vi "carica dati prove.vi"(4 "Riga selezionata":i32, 6 "TIPO COLLEGAMENTO":u16, 7 "Carica tabelle?":bool, 8 "Dati in":string[][](array[string]), 9 "Tabella":i32, 10 "prova":string, 11 "Dati prove in":T1) -> (0 "Per tabella":string[][](array[string]), 1 "Riga selezionata":string[](array[string]), 3 "Dati prove out":T1)   [LabVIEW 2019]
uses:
  TypeDef/Dati collaudo.ctl
panel:
  out "x-y":u32
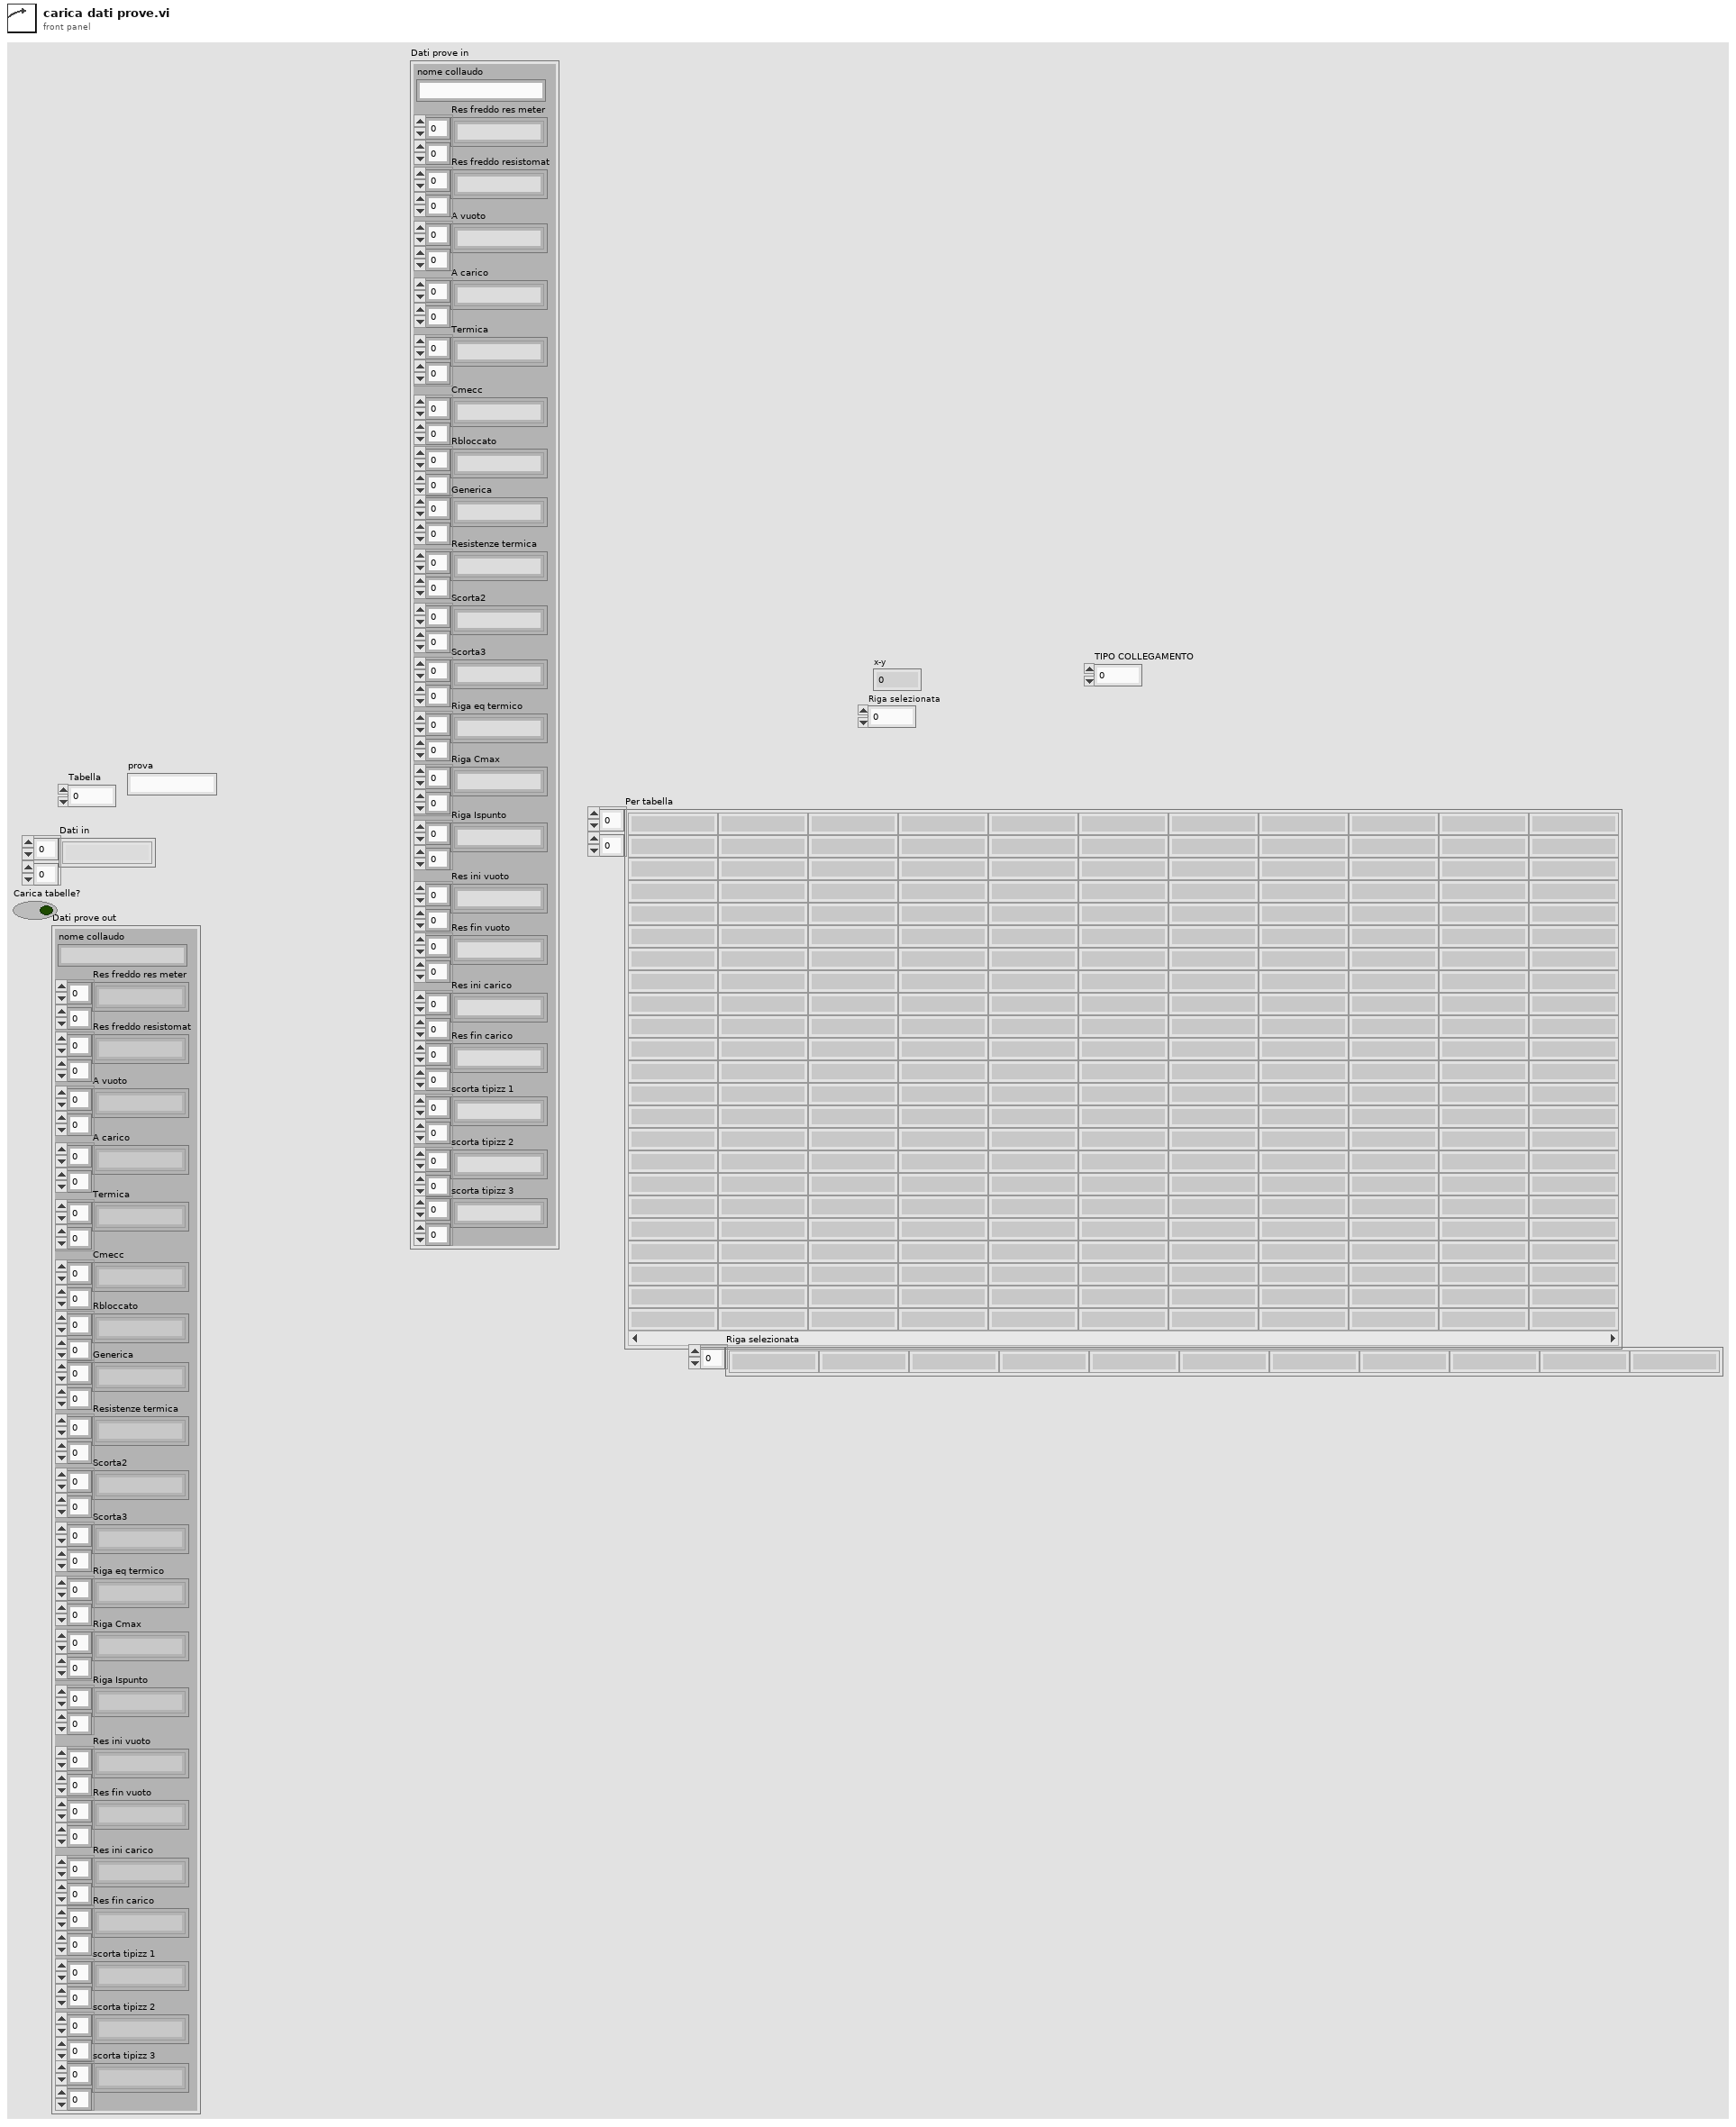
[diagram p1: front panel]
types:
  T1 = typedef "Dati collaudo.ctl" = cluster{"nome collaudo":string, "Res freddo res meter":string[][], "Res freddo resistomat":string[][], "A vuoto":string[][], "A carico":string[][], "Termica":string[][], "Cmecc":string[][], "Rbloccato":string[][], "Generica":string[][], "Resistenze termica":string[][], "Scorta2":string[][], "Scorta3":string[][], "Riga eq termico":string[][], "Riga Cmax":string[][], "Riga Ispunto":string[][], "Res ini vuoto":string[][], "Res fin vuoto":string[][], "Res ini carico":string[][], "Res fin carico":string[][], "scorta tipizz 1":string[][], "scorta tipizz 2":string[][], "scorta tipizz 3":string[][]}
  T2 = cluster{"Nome":string, "TAB":cluster{"Visibile ?":bool, "Salva?":bool}, "decimali":i8, "Medie RT":i8}[]
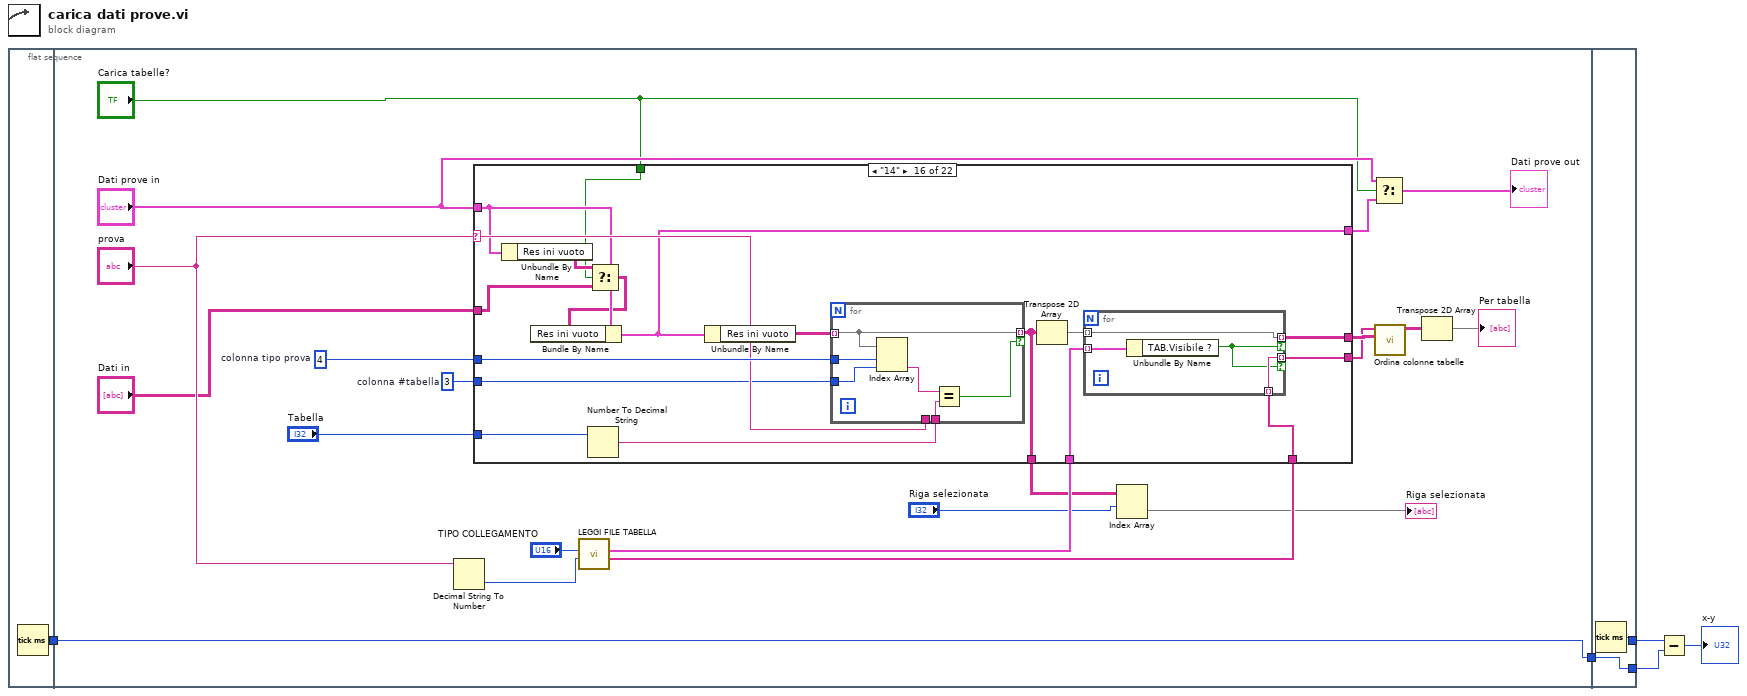
[diagram p0: block diagram]
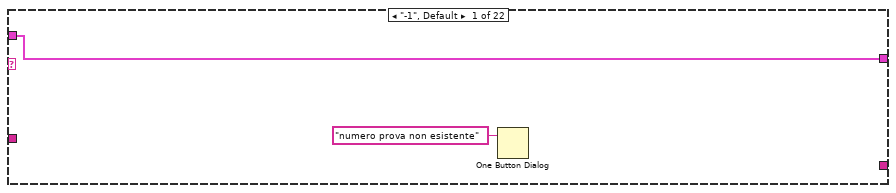
[diagram p2: hidden frame]
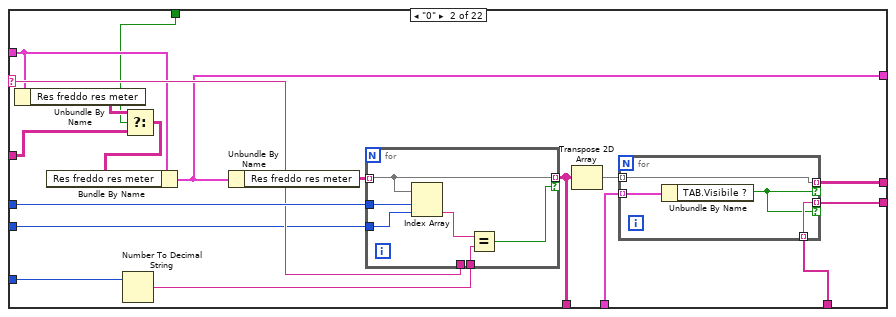
[diagram p3: hidden frame]
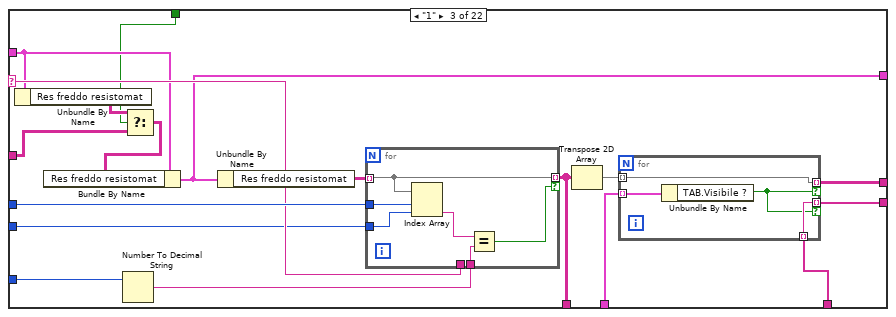
[diagram p4: hidden frame]
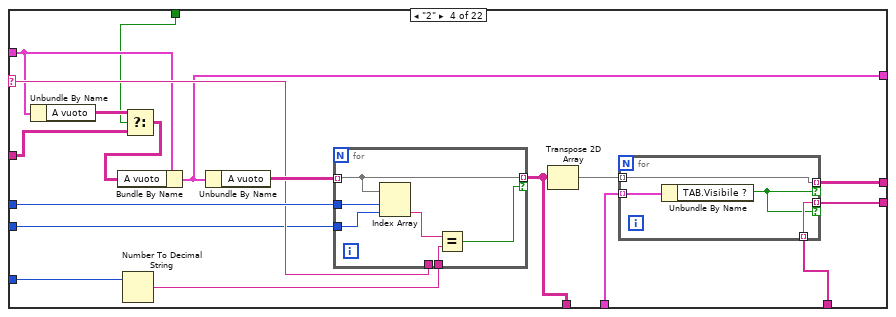
[diagram p5: hidden frame]
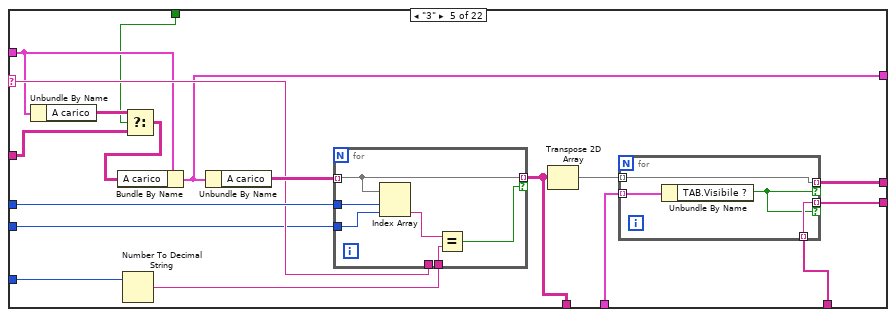
[diagram p6: hidden frame]
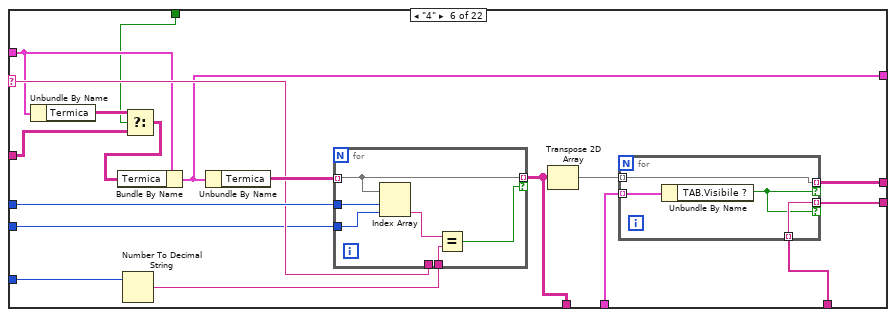
[diagram p7: hidden frame]
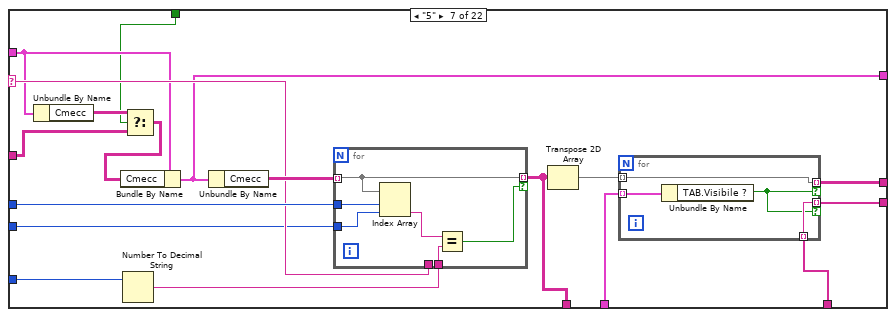
[diagram p8: hidden frame]
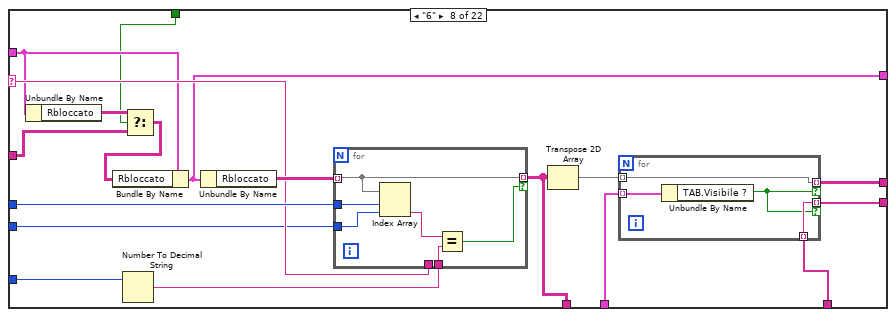
[diagram p9: hidden frame]
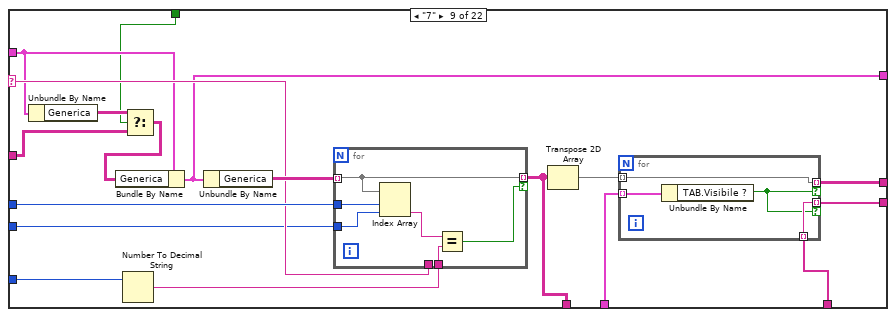
[diagram p10: hidden frame]
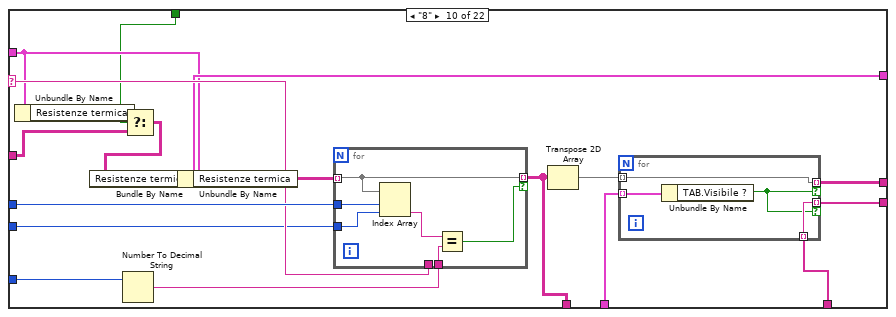
[diagram p11: hidden frame]
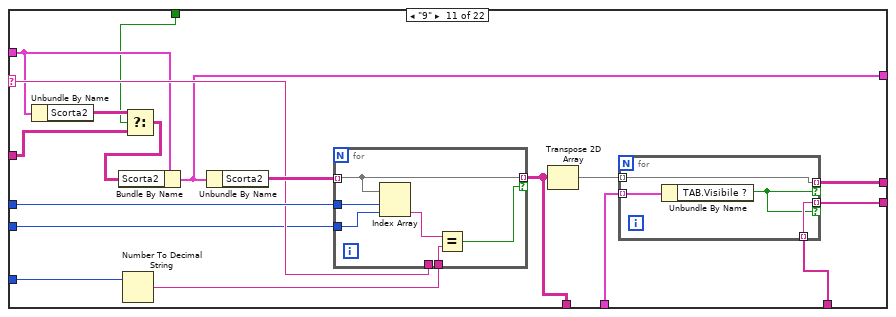
[diagram p12: hidden frame]
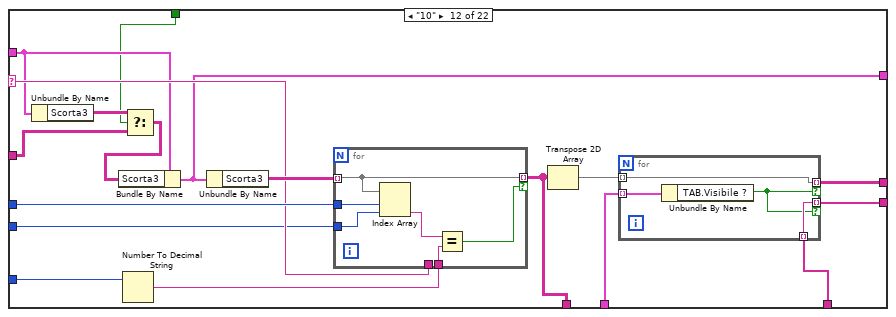
[diagram p13: hidden frame]
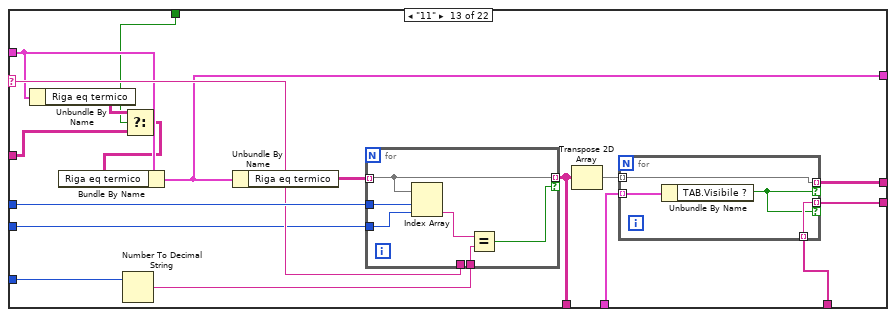
[diagram p14: hidden frame]
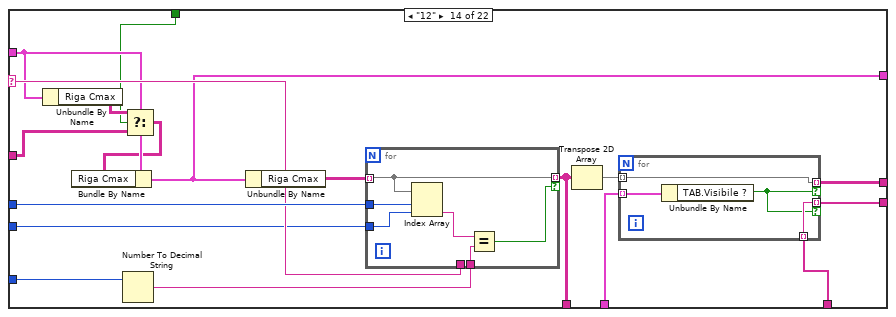
[diagram p15: hidden frame]
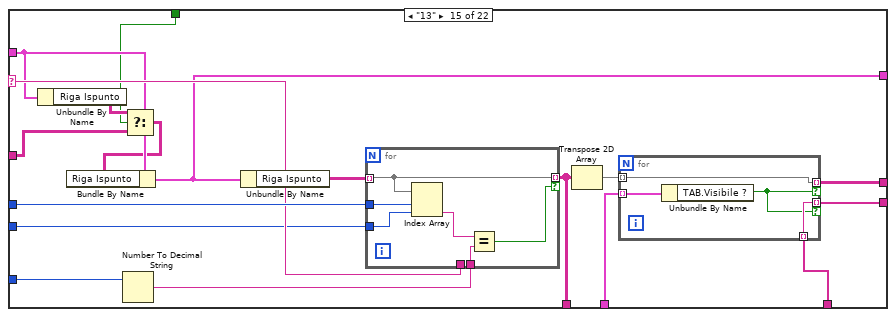
[diagram p16: hidden frame]
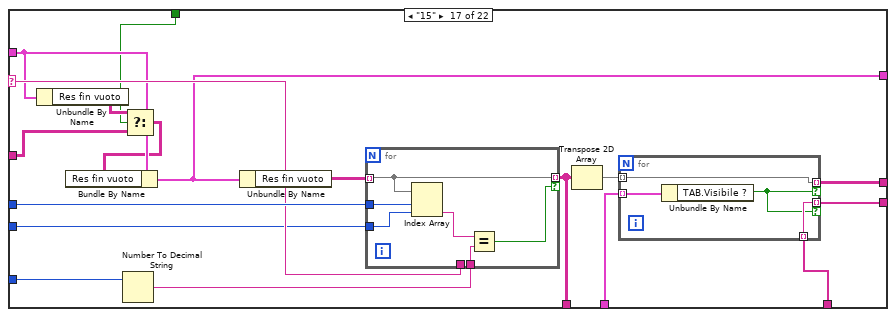
[diagram p17: hidden frame]
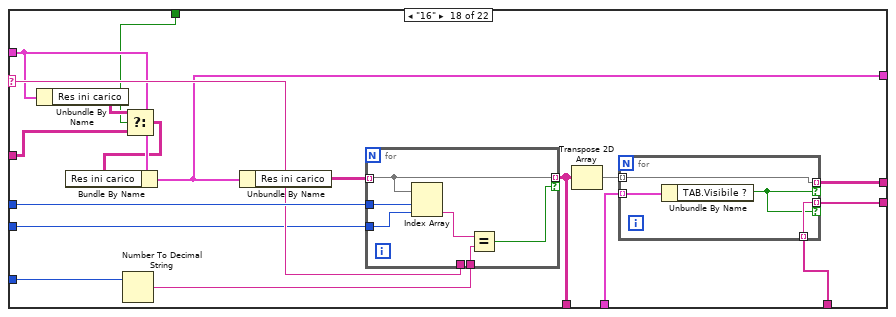
[diagram p18: hidden frame]
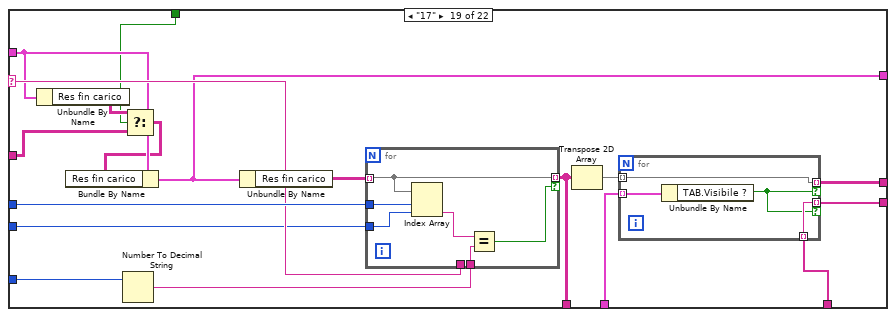
[diagram p19: hidden frame]
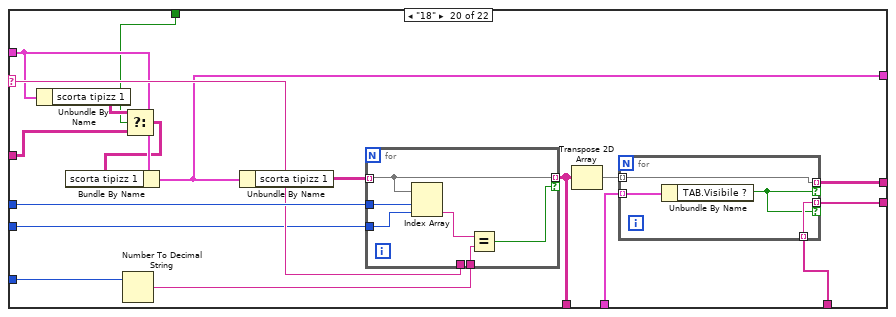
[diagram p20: hidden frame]
diagram:
  n1 = flat-sequence {
    tunnel: [w6] -> w2
    tunnel: [w13] -> w3
    tunnel: w2 -> [w13]
    tunnel: [w619] -> w5
    tunnel: [w618] -> w4
    tunnel: w3 -> [w618]
    frame #0 {
      n2 = Tick Count (ms)() -> (millisecond timer value=w6:u32)
    }
    frame #1 {
      w19 = 3  # colonna #tabella
      w20 = 4  # colonna tipo prova
      n3 = Decimal String To Number(string="prova") -> (number=w14:i32)  [unwired: 2 in, 1 out]
      n4 = call "LEGGI FILE TABELLA.vi"("INDICE TABELLA"=w14, "TIPO COLLEGAMENTO"="TIPO COLLEGAMENTO") -> ("Array INDICI"=w16:string[], "Array"=w17:T2)  [unwired: 7 in, 1 out]
      n5 = case shown="\"14\"" "prova" {
        selector: "prova" -> [_ w41 w69 w97 w125 w153 w181 w209 w237 w265 w293 w321 w349 w377 w405 w433 w461 w489 w517 w545 w573 w601]
        tunnel: "Dati prove in" -> [w29 w34 w62 w90 w118 w146 w174 w202 w230 w258 w286 w314 w342 w370 w398 w426 w454 w482 w510 w538 w566 w594]
        tunnel: [w29 w40 w68 w96 w124 w152 w180 w208 w236 w264 w292 w320 w348 w376 w404 w432 w460 w488 w516 w544 w572 w600] -> w26
        tunnel: "Tabella" -> [_ w39 w67 w95 w123 w151 w179 w207 w235 w263 w291 w319 w347 w375 w403 w431 w459 w487 w515 w543 w571 w599]
        tunnel: [_ w47 w75 w103 w131 w159 w187 w215 w243 w271 w299 w327 w355 w383 w411 w439 w467 w495 w523 w551 w579 w607] -> w23
        tunnel: w16 -> [_ w45 w73 w101 w129 w157 w185 w213 w241 w269 w297 w325 w353 w381 w409 w437 w465 w493 w521 w549 w577 w605]
        tunnel: [_ w44 w72 w100 w128 w156 w184 w212 w240 w268 w296 w324 w352 w380 w408 w436 w464 w492 w520 w548 w576 w604] -> w21
        tunnel: w20 -> [_ w42 w70 w98 w126 w154 w182 w210 w238 w266 w294 w322 w350 w378 w406 w434 w462 w490 w518 w546 w574 w602]
        tunnel: w19 -> [_ w38 w66 w94 w122 w150 w178 w206 w234 w262 w290 w318 w346 w374 w402 w430 w458 w486 w514 w542 w570 w598]
        tunnel: w17 -> [_ w36 w64 w92 w120 w148 w176 w204 w232 w260 w288 w316 w344 w372 w400 w428 w456 w484 w512 w540 w568 w596]
        tunnel: "Carica tabelle?" -> [_ w32 w60 w88 w116 w144 w172 w200 w228 w256 w284 w312 w340 w368 w396 w424 w452 w480 w508 w536 w564 w592]
        tunnel: "Dati in" -> [_ w33 w61 w89 w117 w145 w173 w201 w229 w257 w285 w313 w341 w369 w397 w425 w453 w481 w509 w537 w565 w593]
        tunnel: [_ w30 w58 w86 w114 w142 w170 w198 w226 w254 w282 w310 w338 w366 w394 w422 w450 w478 w506 w534 w562 w590] -> w9
        frame "-1", Default {
          n6 = One Button Dialog(message="numero prova non esistente") -> ()  [unwired: 1 in, 1 out]
        }
        frame "0" {
          n7 = Unbundle By Name(w34) -> ("Res freddo res meter"=w35:string[][])
          n8 = Number To Decimal String(number=w39) -> (decimal integer string=w37:string)  [unwired: 1 in]
          n9 = Select(t=w35, s=w32, f=w33) -> (s? t:f=w31:string[][])
          n10 = Bundle By Name(cluster=w34, "Res freddo res meter"=w31) -> (w40:T1)
          n11 = Unbundle By Name(w40) -> ("Res freddo res meter"=w43:string[][])
          n12 = for {
            tunnel: w43 -> [w52] mode=indexing
            tunnel: [w52] -> w30 mode=indexing if=w48
            tunnel: w42 -> [w53]
            tunnel: w41 -> [_]
            tunnel: w38 -> [w51]
            tunnel: w37 -> [w49]
            n13 = Index Array(array=w52, index #1=w53, index #2=w51) -> (element #2=w50:string)  [unwired: 1 out]
            n14 = Equal?(x=w50, y=w49) -> (x = y?=w48:bool)
          }
          n15 = Transpose 2D Array(2D array=w30) -> (transposed array=w46:string[][])
          n16 = for {
            tunnel: w46 -> [w57] mode=indexing
            tunnel: [w57] -> w47 mode=indexing if=w54
            tunnel: w36 -> [w56] mode=indexing
            tunnel: [w55] -> w44 mode=indexing if=w54
            tunnel: w45 -> [w55] mode=indexing
            n17 = Unbundle By Name(w56) -> ("TAB.Visibile ?"=w54:bool)
          }
        }
        frame "1" {
          n18 = Unbundle By Name(w62) -> ("Res freddo resistomat"=w63:string[][])
          n19 = Number To Decimal String(number=w67) -> (decimal integer string=w65:string)  [unwired: 1 in]
          n20 = Select(t=w63, s=w60, f=w61) -> (s? t:f=w59:string[][])
          n21 = Bundle By Name(cluster=w62, "Res freddo resistomat"=w59) -> (w68:T1)
          n22 = Unbundle By Name(w68) -> ("Res freddo resistomat"=w71:string[][])
          n23 = for {
            tunnel: w71 -> [w80] mode=indexing
            tunnel: [w80] -> w58 mode=indexing if=w76
            tunnel: w70 -> [w81]
            tunnel: w69 -> [_]
            tunnel: w66 -> [w79]
            tunnel: w65 -> [w77]
            n24 = Index Array(array=w80, index #1=w81, index #2=w79) -> (element #2=w78:string)  [unwired: 1 out]
            n25 = Equal?(x=w78, y=w77) -> (x = y?=w76:bool)
          }
          n26 = Transpose 2D Array(2D array=w58) -> (transposed array=w74:string[][])
          n27 = for {
            tunnel: w74 -> [w85] mode=indexing
            tunnel: [w85] -> w75 mode=indexing if=w82
            tunnel: w64 -> [w84] mode=indexing
            tunnel: [w83] -> w72 mode=indexing if=w82
            tunnel: w73 -> [w83] mode=indexing
            n28 = Unbundle By Name(w84) -> ("TAB.Visibile ?"=w82:bool)
          }
        }
        frame "2" {
          n29 = Unbundle By Name(w90) -> ("A vuoto"=w91:string[][])
          n30 = Number To Decimal String(number=w95) -> (decimal integer string=w93:string)  [unwired: 1 in]
          n31 = Select(t=w91, s=w88, f=w89) -> (s? t:f=w87:string[][])
          n32 = Bundle By Name(cluster=w90, "A vuoto"=w87) -> (w96:T1)
          n33 = Unbundle By Name(w96) -> ("A vuoto"=w99:string[][])
          n34 = for {
            tunnel: w99 -> [w108] mode=indexing
            tunnel: [w108] -> w86 mode=indexing if=w104
            tunnel: w98 -> [w109]
            tunnel: w97 -> [_]
            tunnel: w94 -> [w107]
            tunnel: w93 -> [w105]
            n35 = Index Array(array=w108, index #1=w109, index #2=w107) -> (element #2=w106:string)  [unwired: 1 out]
            n36 = Equal?(x=w106, y=w105) -> (x = y?=w104:bool)
          }
          n37 = Transpose 2D Array(2D array=w86) -> (transposed array=w102:string[][])
          n38 = for {
            tunnel: w102 -> [w113] mode=indexing
            tunnel: [w113] -> w103 mode=indexing if=w110
            tunnel: w92 -> [w112] mode=indexing
            tunnel: [w111] -> w100 mode=indexing if=w110
            tunnel: w101 -> [w111] mode=indexing
            n39 = Unbundle By Name(w112) -> ("TAB.Visibile ?"=w110:bool)
          }
        }
        frame "3" {
          n40 = Unbundle By Name(w118) -> ("A carico"=w119:string[][])
          n41 = Number To Decimal String(number=w123) -> (decimal integer string=w121:string)  [unwired: 1 in]
          n42 = Select(t=w119, s=w116, f=w117) -> (s? t:f=w115:string[][])
          n43 = Bundle By Name(cluster=w118, "A carico"=w115) -> (w124:T1)
          n44 = Unbundle By Name(w124) -> ("A carico"=w127:string[][])
          n45 = for {
            tunnel: w127 -> [w136] mode=indexing
            tunnel: [w136] -> w114 mode=indexing if=w132
            tunnel: w126 -> [w137]
            tunnel: w125 -> [_]
            tunnel: w122 -> [w135]
            tunnel: w121 -> [w133]
            n46 = Index Array(array=w136, index #1=w137, index #2=w135) -> (element #2=w134:string)  [unwired: 1 out]
            n47 = Equal?(x=w134, y=w133) -> (x = y?=w132:bool)
          }
          n48 = Transpose 2D Array(2D array=w114) -> (transposed array=w130:string[][])
          n49 = for {
            tunnel: w130 -> [w141] mode=indexing
            tunnel: [w141] -> w131 mode=indexing if=w138
            tunnel: w120 -> [w140] mode=indexing
            tunnel: [w139] -> w128 mode=indexing if=w138
            tunnel: w129 -> [w139] mode=indexing
            n50 = Unbundle By Name(w140) -> ("TAB.Visibile ?"=w138:bool)
          }
        }
        frame "4" {
          n51 = Unbundle By Name(w146) -> ("Termica"=w147:string[][])
          n52 = Number To Decimal String(number=w151) -> (decimal integer string=w149:string)  [unwired: 1 in]
          n53 = Select(t=w147, s=w144, f=w145) -> (s? t:f=w143:string[][])
          n54 = Bundle By Name(cluster=w146, "Termica"=w143) -> (w152:T1)
          n55 = Unbundle By Name(w152) -> ("Termica"=w155:string[][])
          n56 = for {
            tunnel: w155 -> [w164] mode=indexing
            tunnel: [w164] -> w142 mode=indexing if=w160
            tunnel: w154 -> [w165]
            tunnel: w153 -> [_]
            tunnel: w150 -> [w163]
            tunnel: w149 -> [w161]
            n57 = Index Array(array=w164, index #1=w165, index #2=w163) -> (element #2=w162:string)  [unwired: 1 out]
            n58 = Equal?(x=w162, y=w161) -> (x = y?=w160:bool)
          }
          n59 = Transpose 2D Array(2D array=w142) -> (transposed array=w158:string[][])
          n60 = for {
            tunnel: w158 -> [w169] mode=indexing
            tunnel: [w169] -> w159 mode=indexing if=w166
            tunnel: w148 -> [w168] mode=indexing
            tunnel: [w167] -> w156 mode=indexing if=w166
            tunnel: w157 -> [w167] mode=indexing
            n61 = Unbundle By Name(w168) -> ("TAB.Visibile ?"=w166:bool)
          }
        }
        frame "5" {
          n62 = Unbundle By Name(w174) -> ("Cmecc"=w175:string[][])
          n63 = Number To Decimal String(number=w179) -> (decimal integer string=w177:string)  [unwired: 1 in]
          n64 = Select(t=w175, s=w172, f=w173) -> (s? t:f=w171:string[][])
          n65 = Bundle By Name(cluster=w174, "Cmecc"=w171) -> (w180:T1)
          n66 = Unbundle By Name(w180) -> ("Cmecc"=w183:string[][])
          n67 = for {
            tunnel: w183 -> [w192] mode=indexing
            tunnel: [w192] -> w170 mode=indexing if=w188
            tunnel: w182 -> [w193]
            tunnel: w181 -> [_]
            tunnel: w178 -> [w191]
            tunnel: w177 -> [w189]
            n68 = Index Array(array=w192, index #1=w193, index #2=w191) -> (element #2=w190:string)  [unwired: 1 out]
            n69 = Equal?(x=w190, y=w189) -> (x = y?=w188:bool)
          }
          n70 = Transpose 2D Array(2D array=w170) -> (transposed array=w186:string[][])
          n71 = for {
            tunnel: w186 -> [w197] mode=indexing
            tunnel: [w197] -> w187 mode=indexing if=w194
            tunnel: w176 -> [w196] mode=indexing
            tunnel: [w195] -> w184 mode=indexing if=w194
            tunnel: w185 -> [w195] mode=indexing
            n72 = Unbundle By Name(w196) -> ("TAB.Visibile ?"=w194:bool)
          }
        }
        frame "6" {
          n73 = Unbundle By Name(w202) -> ("Rbloccato"=w203:string[][])
          n74 = Number To Decimal String(number=w207) -> (decimal integer string=w205:string)  [unwired: 1 in]
          n75 = Select(t=w203, s=w200, f=w201) -> (s? t:f=w199:string[][])
          n76 = Bundle By Name(cluster=w202, "Rbloccato"=w199) -> (w208:T1)
          n77 = Unbundle By Name(w208) -> ("Rbloccato"=w211:string[][])
          n78 = for {
            tunnel: w211 -> [w220] mode=indexing
            tunnel: [w220] -> w198 mode=indexing if=w216
            tunnel: w210 -> [w221]
            tunnel: w209 -> [_]
            tunnel: w206 -> [w219]
            tunnel: w205 -> [w217]
            n79 = Index Array(array=w220, index #1=w221, index #2=w219) -> (element #2=w218:string)  [unwired: 1 out]
            n80 = Equal?(x=w218, y=w217) -> (x = y?=w216:bool)
          }
          n81 = Transpose 2D Array(2D array=w198) -> (transposed array=w214:string[][])
          n82 = for {
            tunnel: w214 -> [w225] mode=indexing
            tunnel: [w225] -> w215 mode=indexing if=w222
            tunnel: w204 -> [w224] mode=indexing
            tunnel: [w223] -> w212 mode=indexing if=w222
            tunnel: w213 -> [w223] mode=indexing
            n83 = Unbundle By Name(w224) -> ("TAB.Visibile ?"=w222:bool)
          }
        }
        frame "7" {
          n84 = Unbundle By Name(w230) -> ("Generica"=w231:string[][])
          n85 = Number To Decimal String(number=w235) -> (decimal integer string=w233:string)  [unwired: 1 in]
          n86 = Select(t=w231, s=w228, f=w229) -> (s? t:f=w227:string[][])
          n87 = Bundle By Name(cluster=w230, "Generica"=w227) -> (w236:T1)
          n88 = Unbundle By Name(w236) -> ("Generica"=w239:string[][])
          n89 = for {
            tunnel: w239 -> [w248] mode=indexing
            tunnel: [w248] -> w226 mode=indexing if=w244
            tunnel: w238 -> [w249]
            tunnel: w237 -> [_]
            tunnel: w234 -> [w247]
            tunnel: w233 -> [w245]
            n90 = Index Array(array=w248, index #1=w249, index #2=w247) -> (element #2=w246:string)  [unwired: 1 out]
            n91 = Equal?(x=w246, y=w245) -> (x = y?=w244:bool)
          }
          n92 = Transpose 2D Array(2D array=w226) -> (transposed array=w242:string[][])
          n93 = for {
            tunnel: w242 -> [w253] mode=indexing
            tunnel: [w253] -> w243 mode=indexing if=w250
            tunnel: w232 -> [w252] mode=indexing
            tunnel: [w251] -> w240 mode=indexing if=w250
            tunnel: w241 -> [w251] mode=indexing
            n94 = Unbundle By Name(w252) -> ("TAB.Visibile ?"=w250:bool)
          }
        }
        frame "8" {
          n95 = Unbundle By Name(w258) -> ("Resistenze termica"=w259:string[][])
          n96 = Number To Decimal String(number=w263) -> (decimal integer string=w261:string)  [unwired: 1 in]
          n97 = Select(t=w259, s=w256, f=w257) -> (s? t:f=w255:string[][])
          n98 = Bundle By Name(cluster=w258, "Resistenze termica"=w255) -> (w264:T1)
          n99 = Unbundle By Name(w264) -> ("Resistenze termica"=w267:string[][])
          n100 = for {
            tunnel: w267 -> [w276] mode=indexing
            tunnel: [w276] -> w254 mode=indexing if=w272
            tunnel: w266 -> [w277]
            tunnel: w265 -> [_]
            tunnel: w262 -> [w275]
            tunnel: w261 -> [w273]
            n101 = Index Array(array=w276, index #1=w277, index #2=w275) -> (element #2=w274:string)  [unwired: 1 out]
            n102 = Equal?(x=w274, y=w273) -> (x = y?=w272:bool)
          }
          n103 = Transpose 2D Array(2D array=w254) -> (transposed array=w270:string[][])
          n104 = for {
            tunnel: w270 -> [w281] mode=indexing
            tunnel: [w281] -> w271 mode=indexing if=w278
            tunnel: w260 -> [w280] mode=indexing
            tunnel: [w279] -> w268 mode=indexing if=w278
            tunnel: w269 -> [w279] mode=indexing
            n105 = Unbundle By Name(w280) -> ("TAB.Visibile ?"=w278:bool)
          }
        }
        frame "9" {
          n106 = Unbundle By Name(w286) -> ("Scorta2"=w287:string[][])
          n107 = Number To Decimal String(number=w291) -> (decimal integer string=w289:string)  [unwired: 1 in]
          n108 = Select(t=w287, s=w284, f=w285) -> (s? t:f=w283:string[][])
          n109 = Bundle By Name(cluster=w286, "Scorta2"=w283) -> (w292:T1)
          n110 = Unbundle By Name(w292) -> ("Scorta2"=w295:string[][])
          n111 = for {
            tunnel: w295 -> [w304] mode=indexing
            tunnel: [w304] -> w282 mode=indexing if=w300
            tunnel: w294 -> [w305]
            tunnel: w293 -> [_]
            tunnel: w290 -> [w303]
            tunnel: w289 -> [w301]
            n112 = Index Array(array=w304, index #1=w305, index #2=w303) -> (element #2=w302:string)  [unwired: 1 out]
            n113 = Equal?(x=w302, y=w301) -> (x = y?=w300:bool)
          }
          n114 = Transpose 2D Array(2D array=w282) -> (transposed array=w298:string[][])
          n115 = for {
            tunnel: w298 -> [w309] mode=indexing
            tunnel: [w309] -> w299 mode=indexing if=w306
            tunnel: w288 -> [w308] mode=indexing
            tunnel: [w307] -> w296 mode=indexing if=w306
            tunnel: w297 -> [w307] mode=indexing
            n116 = Unbundle By Name(w308) -> ("TAB.Visibile ?"=w306:bool)
          }
        }
        frame "10" {
          n117 = Unbundle By Name(w314) -> ("Scorta3"=w315:string[][])
          n118 = Number To Decimal String(number=w319) -> (decimal integer string=w317:string)  [unwired: 1 in]
          n119 = Select(t=w315, s=w312, f=w313) -> (s? t:f=w311:string[][])
          n120 = Bundle By Name(cluster=w314, "Scorta3"=w311) -> (w320:T1)
          n121 = Unbundle By Name(w320) -> ("Scorta3"=w323:string[][])
          n122 = for {
            tunnel: w323 -> [w332] mode=indexing
            tunnel: [w332] -> w310 mode=indexing if=w328
            tunnel: w322 -> [w333]
            tunnel: w321 -> [_]
            tunnel: w318 -> [w331]
            tunnel: w317 -> [w329]
            n123 = Index Array(array=w332, index #1=w333, index #2=w331) -> (element #2=w330:string)  [unwired: 1 out]
            n124 = Equal?(x=w330, y=w329) -> (x = y?=w328:bool)
          }
          n125 = Transpose 2D Array(2D array=w310) -> (transposed array=w326:string[][])
          n126 = for {
            tunnel: w326 -> [w337] mode=indexing
            tunnel: [w337] -> w327 mode=indexing if=w334
            tunnel: w316 -> [w336] mode=indexing
            tunnel: [w335] -> w324 mode=indexing if=w334
            tunnel: w325 -> [w335] mode=indexing
            n127 = Unbundle By Name(w336) -> ("TAB.Visibile ?"=w334:bool)
          }
        }
        frame "11" {
          n128 = Unbundle By Name(w342) -> ("Riga eq termico"=w343:string[][])
          n129 = Number To Decimal String(number=w347) -> (decimal integer string=w345:string)  [unwired: 1 in]
          n130 = Select(t=w343, s=w340, f=w341) -> (s? t:f=w339:string[][])
          n131 = Bundle By Name(cluster=w342, "Riga eq termico"=w339) -> (w348:T1)
          n132 = Unbundle By Name(w348) -> ("Riga eq termico"=w351:string[][])
          n133 = for {
            tunnel: w351 -> [w360] mode=indexing
            tunnel: [w360] -> w338 mode=indexing if=w356
            tunnel: w350 -> [w361]
            tunnel: w349 -> [_]
            tunnel: w346 -> [w359]
            tunnel: w345 -> [w357]
            n134 = Index Array(array=w360, index #1=w361, index #2=w359) -> (element #2=w358:string)  [unwired: 1 out]
            n135 = Equal?(x=w358, y=w357) -> (x = y?=w356:bool)
          }
          n136 = Transpose 2D Array(2D array=w338) -> (transposed array=w354:string[][])
          n137 = for {
            tunnel: w354 -> [w365] mode=indexing
            tunnel: [w365] -> w355 mode=indexing if=w362
            tunnel: w344 -> [w364] mode=indexing
            tunnel: [w363] -> w352 mode=indexing if=w362
            tunnel: w353 -> [w363] mode=indexing
            n138 = Unbundle By Name(w364) -> ("TAB.Visibile ?"=w362:bool)
          }
        }
        frame "12" {
          n139 = Unbundle By Name(w370) -> ("Riga Cmax"=w371:string[][])
          n140 = Number To Decimal String(number=w375) -> (decimal integer string=w373:string)  [unwired: 1 in]
          n141 = Select(t=w371, s=w368, f=w369) -> (s? t:f=w367:string[][])
          n142 = Bundle By Name(cluster=w370, "Riga Cmax"=w367) -> (w376:T1)
          n143 = Unbundle By Name(w376) -> ("Riga Cmax"=w379:string[][])
          n144 = for {
            tunnel: w379 -> [w388] mode=indexing
            tunnel: [w388] -> w366 mode=indexing if=w384
            tunnel: w378 -> [w389]
            tunnel: w377 -> [_]
            tunnel: w374 -> [w387]
            tunnel: w373 -> [w385]
            n145 = Index Array(array=w388, index #1=w389, index #2=w387) -> (element #2=w386:string)  [unwired: 1 out]
            n146 = Equal?(x=w386, y=w385) -> (x = y?=w384:bool)
          }
          n147 = Transpose 2D Array(2D array=w366) -> (transposed array=w382:string[][])
          n148 = for {
            tunnel: w382 -> [w393] mode=indexing
            tunnel: [w393] -> w383 mode=indexing if=w390
            tunnel: w372 -> [w392] mode=indexing
            tunnel: [w391] -> w380 mode=indexing if=w390
            tunnel: w381 -> [w391] mode=indexing
            n149 = Unbundle By Name(w392) -> ("TAB.Visibile ?"=w390:bool)
          }
        }
        frame "13" {
          n150 = Unbundle By Name(w398) -> ("Riga Ispunto"=w399:string[][])
          n151 = Number To Decimal String(number=w403) -> (decimal integer string=w401:string)  [unwired: 1 in]
          n152 = Select(t=w399, s=w396, f=w397) -> (s? t:f=w395:string[][])
          n153 = Bundle By Name(cluster=w398, "Riga Ispunto"=w395) -> (w404:T1)
          n154 = Unbundle By Name(w404) -> ("Riga Ispunto"=w407:string[][])
          n155 = for {
            tunnel: w407 -> [w416] mode=indexing
            tunnel: [w416] -> w394 mode=indexing if=w412
            tunnel: w406 -> [w417]
            tunnel: w405 -> [_]
            tunnel: w402 -> [w415]
            tunnel: w401 -> [w413]
            n156 = Index Array(array=w416, index #1=w417, index #2=w415) -> (element #2=w414:string)  [unwired: 1 out]
            n157 = Equal?(x=w414, y=w413) -> (x = y?=w412:bool)
          }
          n158 = Transpose 2D Array(2D array=w394) -> (transposed array=w410:string[][])
          n159 = for {
            tunnel: w410 -> [w421] mode=indexing
            tunnel: [w421] -> w411 mode=indexing if=w418
            tunnel: w400 -> [w420] mode=indexing
            tunnel: [w419] -> w408 mode=indexing if=w418
            tunnel: w409 -> [w419] mode=indexing
            n160 = Unbundle By Name(w420) -> ("TAB.Visibile ?"=w418:bool)
          }
        }
        frame "14" {
          n161 = Unbundle By Name(w426) -> ("Res ini vuoto"=w427:string[][])
          n162 = Number To Decimal String(number=w431) -> (decimal integer string=w429:string)  [unwired: 1 in]
          n163 = Select(t=w427, s=w424, f=w425) -> (s? t:f=w423:string[][])
          n164 = Bundle By Name(cluster=w426, "Res ini vuoto"=w423) -> (w432:T1)
          n165 = Unbundle By Name(w432) -> ("Res ini vuoto"=w435:string[][])
          n166 = for {
            tunnel: w435 -> [w444] mode=indexing
            tunnel: [w444] -> w422 mode=indexing if=w440
            tunnel: w434 -> [w445]
            tunnel: w433 -> [_]
            tunnel: w430 -> [w443]
            tunnel: w429 -> [w441]
            n167 = Index Array(array=w444, index #1=w445, index #2=w443) -> (element #2=w442:string)  [unwired: 1 out]
            n168 = Equal?(x=w442, y=w441) -> (x = y?=w440:bool)
          }
          n169 = Transpose 2D Array(2D array=w422) -> (transposed array=w438:string[][])
          n170 = for {
            tunnel: w438 -> [w449] mode=indexing
            tunnel: [w449] -> w439 mode=indexing if=w446
            tunnel: w428 -> [w448] mode=indexing
            tunnel: [w447] -> w436 mode=indexing if=w446
            tunnel: w437 -> [w447] mode=indexing
            n171 = Unbundle By Name(w448) -> ("TAB.Visibile ?"=w446:bool)
          }
        }
        frame "15" {
          n172 = Unbundle By Name(w454) -> ("Res fin vuoto"=w455:string[][])
          n173 = Number To Decimal String(number=w459) -> (decimal integer string=w457:string)  [unwired: 1 in]
          n174 = Select(t=w455, s=w452, f=w453) -> (s? t:f=w451:string[][])
          n175 = Bundle By Name(cluster=w454, "Res fin vuoto"=w451) -> (w460:T1)
          n176 = Unbundle By Name(w460) -> ("Res fin vuoto"=w463:string[][])
          n177 = for {
            tunnel: w463 -> [w472] mode=indexing
            tunnel: [w472] -> w450 mode=indexing if=w468
            tunnel: w462 -> [w473]
            tunnel: w461 -> [_]
            tunnel: w458 -> [w471]
            tunnel: w457 -> [w469]
            n178 = Index Array(array=w472, index #1=w473, index #2=w471) -> (element #2=w470:string)  [unwired: 1 out]
            n179 = Equal?(x=w470, y=w469) -> (x = y?=w468:bool)
          }
          n180 = Transpose 2D Array(2D array=w450) -> (transposed array=w466:string[][])
          n181 = for {
            tunnel: w466 -> [w477] mode=indexing
            tunnel: [w477] -> w467 mode=indexing if=w474
            tunnel: w456 -> [w476] mode=indexing
            tunnel: [w475] -> w464 mode=indexing if=w474
            tunnel: w465 -> [w475] mode=indexing
            n182 = Unbundle By Name(w476) -> ("TAB.Visibile ?"=w474:bool)
          }
        }
        frame "16" {
          n183 = Unbundle By Name(w482) -> ("Res ini carico"=w483:string[][])
          n184 = Number To Decimal String(number=w487) -> (decimal integer string=w485:string)  [unwired: 1 in]
          n185 = Select(t=w483, s=w480, f=w481) -> (s? t:f=w479:string[][])
          n186 = Bundle By Name(cluster=w482, "Res ini carico"=w479) -> (w488:T1)
          n187 = Unbundle By Name(w488) -> ("Res ini carico"=w491:string[][])
          n188 = for {
            tunnel: w491 -> [w500] mode=indexing
            tunnel: [w500] -> w478 mode=indexing if=w496
            tunnel: w490 -> [w501]
            tunnel: w489 -> [_]
            tunnel: w486 -> [w499]
            tunnel: w485 -> [w497]
            n189 = Index Array(array=w500, index #1=w501, index #2=w499) -> (element #2=w498:string)  [unwired: 1 out]
            n190 = Equal?(x=w498, y=w497) -> (x = y?=w496:bool)
          }
          n191 = Transpose 2D Array(2D array=w478) -> (transposed array=w494:string[][])
          n192 = for {
            tunnel: w494 -> [w505] mode=indexing
            tunnel: [w505] -> w495 mode=indexing if=w502
            tunnel: w484 -> [w504] mode=indexing
            tunnel: [w503] -> w492 mode=indexing if=w502
            tunnel: w493 -> [w503] mode=indexing
            n193 = Unbundle By Name(w504) -> ("TAB.Visibile ?"=w502:bool)
          }
        }
        frame "17" {
          n194 = Unbundle By Name(w510) -> ("Res fin carico"=w511:string[][])
          n195 = Number To Decimal String(number=w515) -> (decimal integer string=w513:string)  [unwired: 1 in]
          n196 = Select(t=w511, s=w508, f=w509) -> (s? t:f=w507:string[][])
          n197 = Bundle By Name(cluster=w510, "Res fin carico"=w507) -> (w516:T1)
          n198 = Unbundle By Name(w516) -> ("Res fin carico"=w519:string[][])
          n199 = for {
            tunnel: w519 -> [w528] mode=indexing
            tunnel: [w528] -> w506 mode=indexing if=w524
            tunnel: w518 -> [w529]
            tunnel: w517 -> [_]
            tunnel: w514 -> [w527]
            tunnel: w513 -> [w525]
            n200 = Index Array(array=w528, index #1=w529, index #2=w527) -> (element #2=w526:string)  [unwired: 1 out]
            n201 = Equal?(x=w526, y=w525) -> (x = y?=w524:bool)
          }
          n202 = Transpose 2D Array(2D array=w506) -> (transposed array=w522:string[][])
          n203 = for {
            tunnel: w522 -> [w533] mode=indexing
            tunnel: [w533] -> w523 mode=indexing if=w530
            tunnel: w512 -> [w532] mode=indexing
            tunnel: [w531] -> w520 mode=indexing if=w530
            tunnel: w521 -> [w531] mode=indexing
            n204 = Unbundle By Name(w532) -> ("TAB.Visibile ?"=w530:bool)
          }
        }
        frame "18" {
          n205 = Unbundle By Name(w538) -> ("scorta tipizz 1"=w539:string[][])
          n206 = Number To Decimal String(number=w543) -> (decimal integer string=w541:string)  [unwired: 1 in]
          n207 = Select(t=w539, s=w536, f=w537) -> (s? t:f=w535:string[][])
          n208 = Bundle By Name(cluster=w538, "scorta tipizz 1"=w535) -> (w544:T1)
          n209 = Unbundle By Name(w544) -> ("scorta tipizz 1"=w547:string[][])
          n210 = for {
            tunnel: w547 -> [w556] mode=indexing
            tunnel: [w556] -> w534 mode=indexing if=w552
            tunnel: w546 -> [w557]
            tunnel: w545 -> [_]
            tunnel: w542 -> [w555]
            tunnel: w541 -> [w553]
            n211 = Index Array(array=w556, index #1=w557, index #2=w555) -> (element #2=w554:string)  [unwired: 1 out]
            n212 = Equal?(x=w554, y=w553) -> (x = y?=w552:bool)
          }
          n213 = Transpose 2D Array(2D array=w534) -> (transposed array=w550:string[][])
          n214 = for {
            tunnel: w550 -> [w561] mode=indexing
            tunnel: [w561] -> w551 mode=indexing if=w558
            tunnel: w540 -> [w560] mode=indexing
            tunnel: [w559] -> w548 mode=indexing if=w558
            tunnel: w549 -> [w559] mode=indexing
            n215 = Unbundle By Name(w560) -> ("TAB.Visibile ?"=w558:bool)
          }
        }
        frame "19" {
          n216 = Unbundle By Name(w566) -> ("scorta tipizz 2"=w567:string[][])
          n217 = Number To Decimal String(number=w571) -> (decimal integer string=w569:string)  [unwired: 1 in]
          n218 = Select(t=w567, s=w564, f=w565) -> (s? t:f=w563:string[][])
          n219 = Bundle By Name(cluster=w566, "scorta tipizz 2"=w563) -> (w572:T1)
          n220 = Unbundle By Name(w572) -> ("scorta tipizz 2"=w575:string[][])
          n221 = for {
            tunnel: w575 -> [w584] mode=indexing
            tunnel: [w584] -> w562 mode=indexing if=w580
            tunnel: w574 -> [w585]
            tunnel: w573 -> [_]
            tunnel: w570 -> [w583]
            tunnel: w569 -> [w581]
            n222 = Index Array(array=w584, index #1=w585, index #2=w583) -> (element #2=w582:string)  [unwired: 1 out]
            n223 = Equal?(x=w582, y=w581) -> (x = y?=w580:bool)
          }
          n224 = Transpose 2D Array(2D array=w562) -> (transposed array=w578:string[][])
          n225 = for {
            tunnel: w578 -> [w589] mode=indexing
            tunnel: [w589] -> w579 mode=indexing if=w586
            tunnel: w568 -> [w588] mode=indexing
            tunnel: [w587] -> w576 mode=indexing if=w586
            tunnel: w577 -> [w587] mode=indexing
            n226 = Unbundle By Name(w588) -> ("TAB.Visibile ?"=w586:bool)
          }
        }
        frame "20" {
          n227 = Unbundle By Name(w594) -> ("scorta tipizz 3"=w595:string[][])
          n228 = Number To Decimal String(number=w599) -> (decimal integer string=w597:string)  [unwired: 1 in]
          n229 = Select(t=w595, s=w592, f=w593) -> (s? t:f=w591:string[][])
          n230 = Bundle By Name(cluster=w594, "scorta tipizz 3"=w591) -> (w600:T1)
          n231 = Unbundle By Name(w600) -> ("scorta tipizz 3"=w603:string[][])
          n232 = for {
            tunnel: w603 -> [w612] mode=indexing
            tunnel: [w612] -> w590 mode=indexing if=w608
            tunnel: w602 -> [w613]
            tunnel: w601 -> [_]
            tunnel: w598 -> [w611]
            tunnel: w597 -> [w609]
            n233 = Index Array(array=w612, index #1=w613, index #2=w611) -> (element #2=w610:string)  [unwired: 1 out]
            n234 = Equal?(x=w610, y=w609) -> (x = y?=w608:bool)
          }
          n235 = Transpose 2D Array(2D array=w590) -> (transposed array=w606:string[][])
          n236 = for {
            tunnel: w606 -> [w617] mode=indexing
            tunnel: [w617] -> w607 mode=indexing if=w614
            tunnel: w596 -> [w616] mode=indexing
            tunnel: [w615] -> w604 mode=indexing if=w614
            tunnel: w605 -> [w615] mode=indexing
            n237 = Unbundle By Name(w616) -> ("TAB.Visibile ?"=w614:bool)
          }
        }
      }
      n238 = Index Array(array=w9, index (row)="Riga selezionata") -> (element=→"Riga selezionata":string[])  [unwired: 1 in]
      n239 = Select(t="Dati prove in", s="Carica tabelle?", f=w26) -> (s? t:f=→"Dati prove out":T1)
      n240 = call "Ordina colonne tabelle.vi"("Array colonne"=w23, "Array indici"=w21) -> ("Array nomi ordinati per inidii"=w22:string[][])  [unwired: 9 in]
      n241 = Transpose 2D Array(2D array=w22) -> (transposed array=→"Per tabella":string[][])
    }
    frame #2 {
      n242 = Tick Count (ms)() -> (millisecond timer value=w619:u32)
    }
  }
  n243 = Subtract(x=w5, y=w4) -> (x-y=→"x-y":u32)
